vi "FTW-TestExecutive-Core_Step_SetStatus.vi"(0 "FTW-TestExecutive-Core In":refnum<class "FTW-TestExecutive-Core.lvclass">, 7 "State":T1, 11 "error in":errorcluster) -> (4 "FTW-TestExecutive-Core Out":refnum<class "FTW-TestExecutive-Core.lvclass">, 15 "error out":errorcluster)   [LabVIEW 2015, in "FTW-TestExecutive-Core.lvclass"]
uses:
  FTW-TestExecutive-Core.lvclass
  FTW-TestExecutive-Step-State.ctl
  FTW-TestExecutive-Core.lvclass/FTW-TestExecutive-Core.ctl
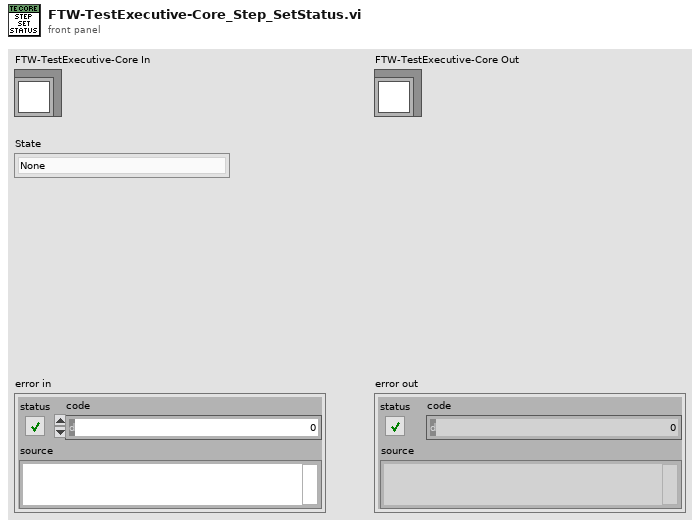
[diagram p1: front panel]
types:
  T1 = typedef "FTW-TestExecutive-Step-State.ctl" = enum8{"None", "Failed", "Passed", "Timed out", "Aborted"}
  T2 = typedef "FTW-TestExecutive-Step.ctl" = cluster{"Name":string, "Type":string, "Path":string, "Config":string, "Elapsed Time":dbl, "Passed":bool, "State":T1, "Results":T3}
  T3 = typedef "FTW-TestExecutive-Results.ctl" = cluster{"Start Time":timestamp, "Elapsed Time":dbl, "Passed":bool}
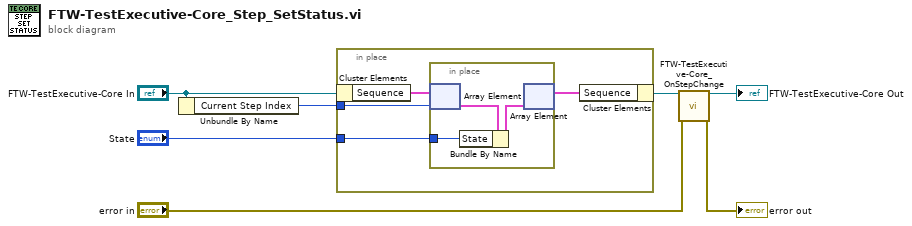
[diagram p0: block diagram]
diagram:
  n1 = Unbundle By Name("FTW-TestExecutive-Core In") -> ("Current Step Index"=w2:i32)
  n2 = in-place {
    in-place-border: w2 -> [w10]
    in-place-border: "State" -> [w8]
    n3 = in-place-cluster #1("FTW-TestExecutive-Core In") -> ("Sequence"=w11:T2[])
    n4 = in-place {
      in-place-border: w8 -> [w12]
      n5 = in-place-array #2(w11, w10) -> (w14:T2)
      n6 = Bundle By Name(cluster=w14, "State"=w12) -> (w13:T2)
      n7 = in-place-array #2(w13) -> (w9:T2[])  [unwired: 1 out]
    }
    n8 = in-place-cluster #1("Sequence"=w9) -> (w3:refnum<class "FTW-TestExecutive-Core.lvclass">)
  }
  n9 = call "FTW-TestExecutive-Core_OnStepChange.vi"("FTW-TestExecutive-Core In"=w3, "error in"="error in") -> ("FTW-TestExecutive-Core Out"=→"FTW-TestExecutive-Core Out":refnum<class "FTW-TestExecutive-Core.lvclass">, "error out"=→"error out":errorcluster)  [unwired: 12 in]
